vi "SELECT many rows Template code.vi"   [LabVIEW 2023, in "SQLite.lvlib"]
doc: "Code template for Preparing an SQL statement and extracting all returned rows."
uses:
  SQLite.lvlib
  SQL Statement.lvclass
  SQL Connection/Connection.lvclass
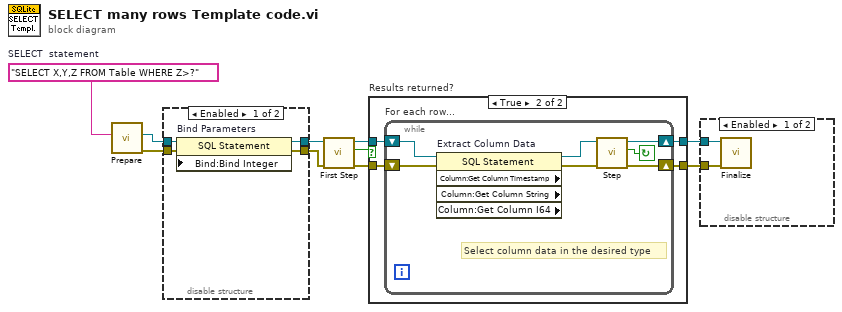
[diagram p0: block diagram]
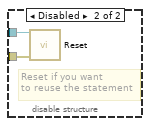
[diagram p2: hidden frame]
diagram:
  w3 = "SELECT X,Y,Z FROM Table WHERE Z>?"  # SELECT  statement
  n1 = call "Prepare.vi"("SQL"=w3) -> ("error out"=w4:errorcluster, "SQL Statement out"=w7:refnum<class "SQL Statement.lvclass">)  [unwired: 6 in, 3 out]
  n2 = disable-structure shown="Enabled" {
    disable-tunnel: w7 -> [w14 w16]
    disable-tunnel: [w13 w16] -> w6
    disable-tunnel: [w12 w15] -> w5
    disable-tunnel: w4 -> [w11 w15]
    frame Enabled {
      n3 = property on="Bind Parameters" class="SQL Statement" props=["Bind:Bind Integer"](reference=w14, error in=w11) -> (reference out=w13:refnum<class "SQL Statement.lvclass">, error out=w12:errorcluster)  [unwired: 1 in]
    }
    frame Disabled {
    }
  }
  n4 = call "First Step.vi"("error in (no error)"=w5, "SQL Statement in"=w6) -> ("error out"=w9:errorcluster, "Row returned"=w10:bool, "SQL Statement out"=w8:refnum<class "SQL Statement.lvclass">)  [unwired: 7 in]
  n5 = case "Results returned?" shown="True" w10 {
    tunnel: [w18 w22] -> w2
    tunnel: [w17 w21] -> w1
    tunnel: w8 -> [w18 w20]
    tunnel: w9 -> [w17 w19]
    frame False {
    }
    frame True {
      n6 = while "For each row..." {
        shift-right: [w28] -> w22
        shift-left: w20 -> [w25]
        shift-right: [w26] -> w21
        shift-left: w19 -> [w24]
        stop <- w23 continue-if-true
        # "Select column data in the desired type"
        n7 = property on="Extract Column Data" class="SQL Statement" props=["Column:Get Column Timestamp", "Column:Get Column String", "Column:Get Column I64"](reference=w25, error in=w24) -> (reference out=w29:refnum<class "SQL Statement.lvclass">, error out=w27:errorcluster)  [unwired: 3 out]
        n8 = call "Step.vi"("error in (no error)"=w27, "SQL Statement in"=w29) -> ("error out"=w26:errorcluster, "Row returned"=w23:bool, "SQL Statement out"=w28:refnum<class "SQL Statement.lvclass">)  [unwired: 7 in]
      }
    }
  }
  n9 = disable-structure shown="Enabled" {
    disable-tunnel: w2 -> [w31 w33]
    disable-tunnel: w1 -> [w30 w32]
    frame Enabled {
      n10 = call "Finalize.vi"("error in (no error)"=w30, "SQL Statement in"=w31) -> ()  [unwired: 9 in, 1 out]
    }
    frame Disabled {
      # "Reset if you want\nto reuse the statement"
      n11 = call "Reset.vi"("error in (no error)"=w32, "SQL Statement in"=w33) -> ()  [unwired: 8 in, 2 out]
    }
  }
